vi "CRYSelect Operator Window Configure.vi"() -> (0 "Selected path":path, 1 "OK State":bool, 3 "Numeric":u16)   [LabVIEW 2013]
uses:
  CRYMainGlobal.vi
  SubVI/CRYMisc vis settings global.vi
panel:
  out "Selected Number":u16
  in  "Cancel":bool
  in  "OK":bool
  out "Mode":bool caption="选择启动配置"
  in  "Mode Selection":u16(ring) items=["None", "2m.ocf", "sig1-scoffft1.ocf"]
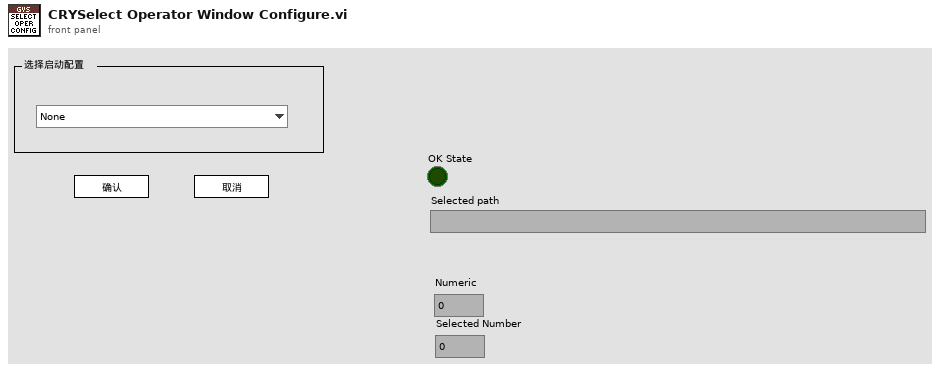
[diagram p1: front panel]
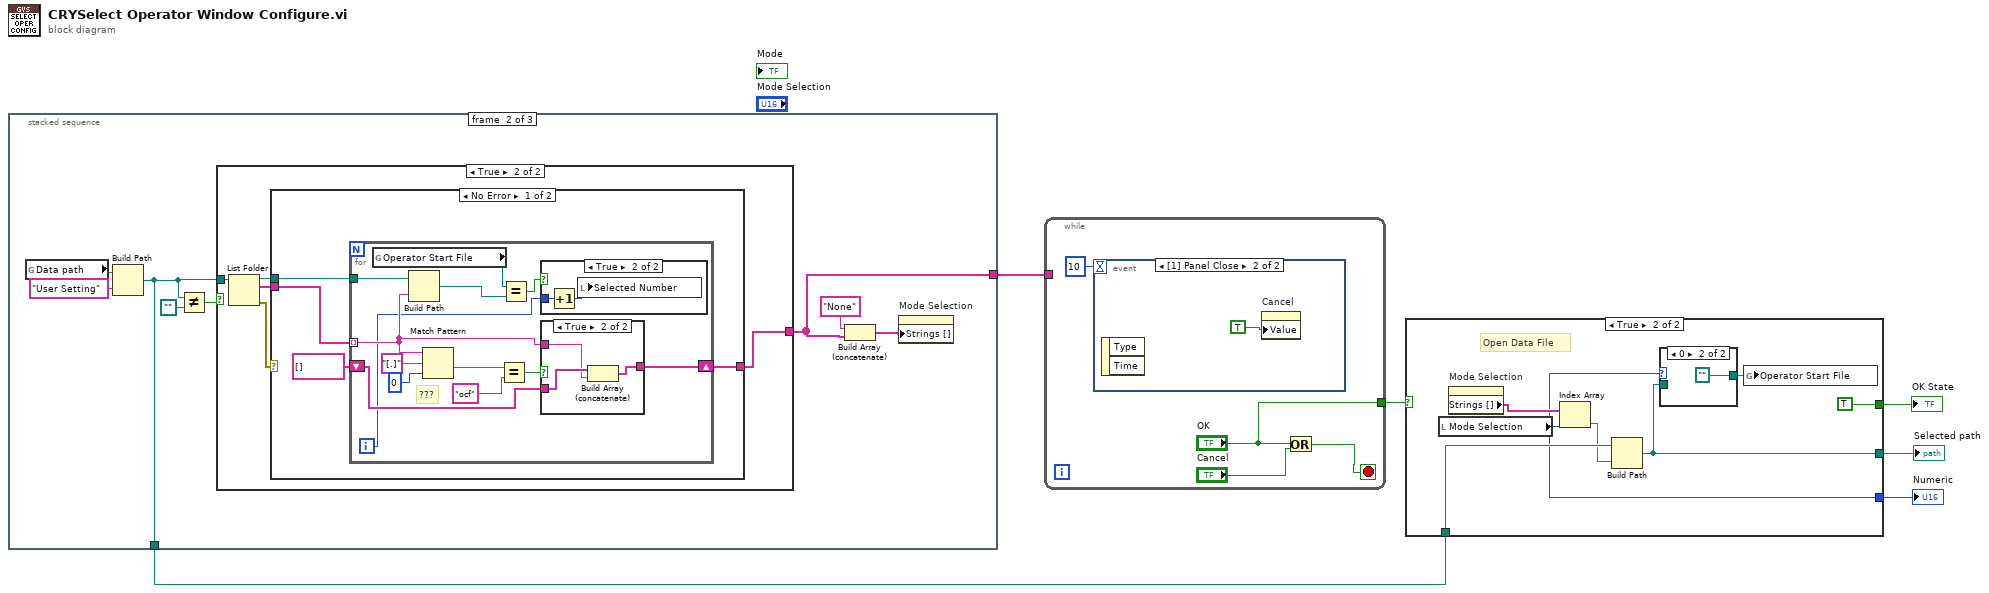
[diagram p0: block diagram]
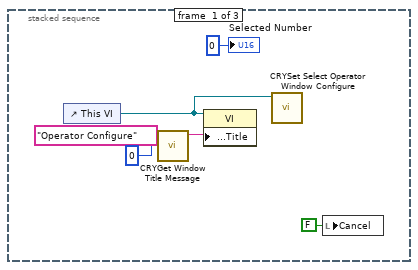
[diagram p2: hidden frame]
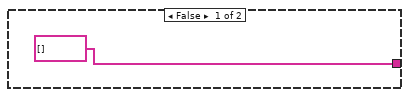
[diagram p3: hidden frame]
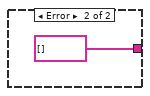
[diagram p6: hidden frame]
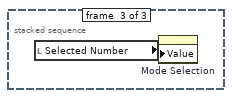
[diagram p7: hidden frame]
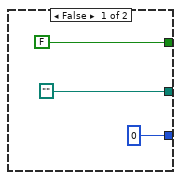
[diagram p8: hidden frame]
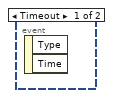
[diagram p10: hidden frame]
diagram:
  n1 = stacked-sequence {
    tunnel: [_ w13 _] -> w6
    tunnel: [_ w16 _] -> w4
    frame #0 {
      n2 = control-ref of="This VI"() -> (w9:refnum<vi>)
      n3 = call "CRYGet Window Title Message.vi"("No"=0, "Kind"="Operator Configure") -> ("Multibyte String"=w10:string)  [unwired: 4 in, 5 out]
      n4 = property class="VI"(reference=w9, "Front Panel.Title"=w10) -> ()  [unwired: 1 in, 2 out]
      n5 = call "CRYSet Select Operator Window Configure.vi"("Vi Ref"=w9) -> ()  [unwired: 11 in]
      n6 = local write "Cancel"(FALSE ("Cancel")) -> ()
      "Selected Number" <- u16 0 ("Selected Number")
    }
    frame #1 {
      n7 = global read "CRYMainGlobal.vi" "Data path"() -> (w17:path)
      n8 = Build Path(base path=w17, name or relative path="User Setting") -> (appended path=w16:path)
      n9 = Not Equal?(x=w16, y=path "") -> (x != y?=w20:bool)
      n10 = case shown="True" w20 {
        tunnel: w16 -> [_ w26]
        tunnel: [string[] [] ("Strings []") w24] -> w13
        frame False {
        }
        frame True {
          n11 = List Folder(path=w26) -> (path out=w22:path, filenames=w25:string[], error out=w23:errorcluster)  [unwired: 1 in, 3 out]
          n12 = case shown="No Error" w23 {
            tunnel: w25 -> [w30 _]
            tunnel: [w28 string[] [] ("file names")] -> w24
            tunnel: w22 -> [w27 _]
            frame No Error {
              n13 = for {
                tunnel: w30 -> [w35] mode=indexing
                shift-right: [w39] -> w28
                shift-left: string[] [] ("file names") -> [w38]
                tunnel: w27 -> [w36]
                i -> [w31]
                # "???"
                n14 = global read "CRYMisc vis settings global.vi" "Operator Start File"() -> (w34:path)
                n15 = Build Path(base path=w36, name or relative path=w35) -> (appended path=w33:path)
                n16 = Match Pattern(string=w35, regular expression="[.]", offset (0)=0) -> (after substring=w37:string)  [unwired: 3 out]
                n17 = Equal?(x=w37, y="ocf") -> (x = y?=w40:bool)
                n18 = Equal?(x=w34, y=w33) -> (x = y?=w32:bool)
                n19 = case shown="True" w32 {
                  tunnel: w31 -> [_ w45]
                  frame False {
                  }
                  frame True {
                    n20 = Increment(x=w45) -> (x+1=w44:i32)
                    n21 = local write "Selected Number"(w44) -> ()
                  }
                }
                n22 = case shown="True" w40 {
                  tunnel: w35 -> [_ w48]
                  tunnel: [w46 w47] -> w39
                  tunnel: w38 -> [w46 w49]
                  frame False {
                  }
                  frame True {
                    n23 = Build Array (concatenate)(w49, w48) -> (w47:string[])
                  }
                }
              }
            }
            frame Error {
            }
          }
        }
      }
      n24 = Build Array (concatenate)("None" ("y"), w13) -> (w14:string[])
      n25 = property on="Mode Selection" class="Ring (strict)"("Strings []"=w14) -> ()  [unwired: 2 in, 2 out]
    }
    frame #2 {
      n26 = local read "Selected Number"() -> (w51:u16)
      n27 = property on="Mode Selection" class="Ring (strict)"("Value"=w51) -> ()  [unwired: 2 in, 2 out]
    }
  }
  n28 = while {
    tunnel: ["OK"] -> w5
    tunnel: w6 -> [_]
    stop <- w54 stop-if-true
    n29 = event shown="[1] Panel Close" {
      selector: _ -> [_ _]
      dyn-events: _ -> [_ _]
      timeout: 10 -> [_ _]
      event Timeout {
        n30 = event-data() -> ()  [unwired: 1 in, 2 out]
      }
      event Panel Close {
        n31 = event-data() -> ()  [unwired: 1 in, 2 out]
        n32 = property on="Cancel" class="Bool (strict)"("Value"=TRUE) -> ()  [unwired: 2 in, 2 out]
      }
    }
    n33 = Or(x="OK", y="Cancel") -> (x .or. y?=w54:bool)
  }
  n34 = case shown="True" w5 {
    tunnel: w4 -> [_ w65]
    tunnel: [FALSE ("OK State") TRUE ("OK State")] -> w3
    tunnel: [path "" w61] -> w2
    tunnel: [u16 0 ("Mode Selection") w62] -> w1
    frame False {
    }
    frame True {
      # "Open Data File"
      n35 = local read "Mode Selection"() -> (w62:u16)
      n36 = property on="Mode Selection" class="Ring (strict)"() -> ("Strings []"=w66:string[])  [unwired: 2 in, 2 out]
      n37 = Index Array(array=w66, index=w62) -> (element=w64:string)
      n38 = Build Path(base path=w65, name or relative path=w64) -> (appended path=w61:path)
      n39 = case shown="0" w62 {
        tunnel: w61 -> [w67 _]
        tunnel: [w67 path ""] -> w60
        frame Default {
        }
        frame 0 {
        }
      }
      n40 = global write "CRYMisc vis settings global.vi" "Operator Start File"(w60) -> ()
    }
  }
  "OK State" <- w3
  "Selected path" <- w2
  "Numeric" <- w1
